vi "WaveSynthV2.vi"(6 "error in":errorcluster) -> (0 "Waves per Pixel":u32, 1 "Delay bw Waves [cycles]":u16, 2 "Sampling Frequency (Hz)":u64, 3 "Waveform":cluster{"tv":dbl[], "DAC Codes":u16[]}, 4 "error out":errorcluster)   [LabVIEW 2018]
uses:
  Controls/WaveFormsAvailable.ctl
  <vilib>/Utility/file.llb/Read Delimited Spreadsheet (DBL).vi
  <vilib>/Utility/file.llb/Write Delimited Spreadsheet (DBL).vi
panel:
  in  "Waveform":T1(tab)
  out "Single Wave":cluster{"all rows":dbl[], "Array":u16[]}(graph)
  out "Wave per Pixel":cluster{dbl[], dbl[]}(graph)
  out "DC Offset":dbl
  out "Frequency Response":cluster{dbl[], dbl[]}(graph)
  in  "Tab Control":enum32{"Temp (Future Controls Idea)", "Page 2"}(tab)
  in  "Scale Precision _Scale":i16(slide)=-3 caption="Scale Precision" scale=-3.0..3.0
  in  "Scale JogWheel":i16(knob) scale=0.0..50.0
  in  "Scale Precision _offset":i16(slide) caption="Scale Precision"
  in  "Offset JogWheel":i16(knob) scale=0.0..50.0
  in  "Scale Precision_Phase":i16(slide) caption="Scale Precision" scale=0.0..3.0
  in  "Phase  JogWheel":i16(knob) scale=0.0..50.0
  out "Time Series":dbl[](array[numeric])
  out "Amplitudes":u16[](array[numeric])
  in  "Save Button":bool
  in  "Start Time (us)":dbl format="%#_6p"
  in  "Number of Samples":u32=2048
  in  "Sampling Frequency (Hz)":u64=1250000000 format="%.2p"
  in  "Waves per Pixel":u32=1
  in  "Delay between waves (us)":dbl
  in  "Frequency (Hz)":u64=40000000 format="%.0p"
  in  "Wave":T2=enum."Ricker"
  in  "Reset Button":bool
  in  "Scale Factor":dbl=1.0
  in  "Offset Factor":dbl
  in  "Phase Delay (Samples)":i32
  in  "Done":bool
  # "Waveform Synthesizer"
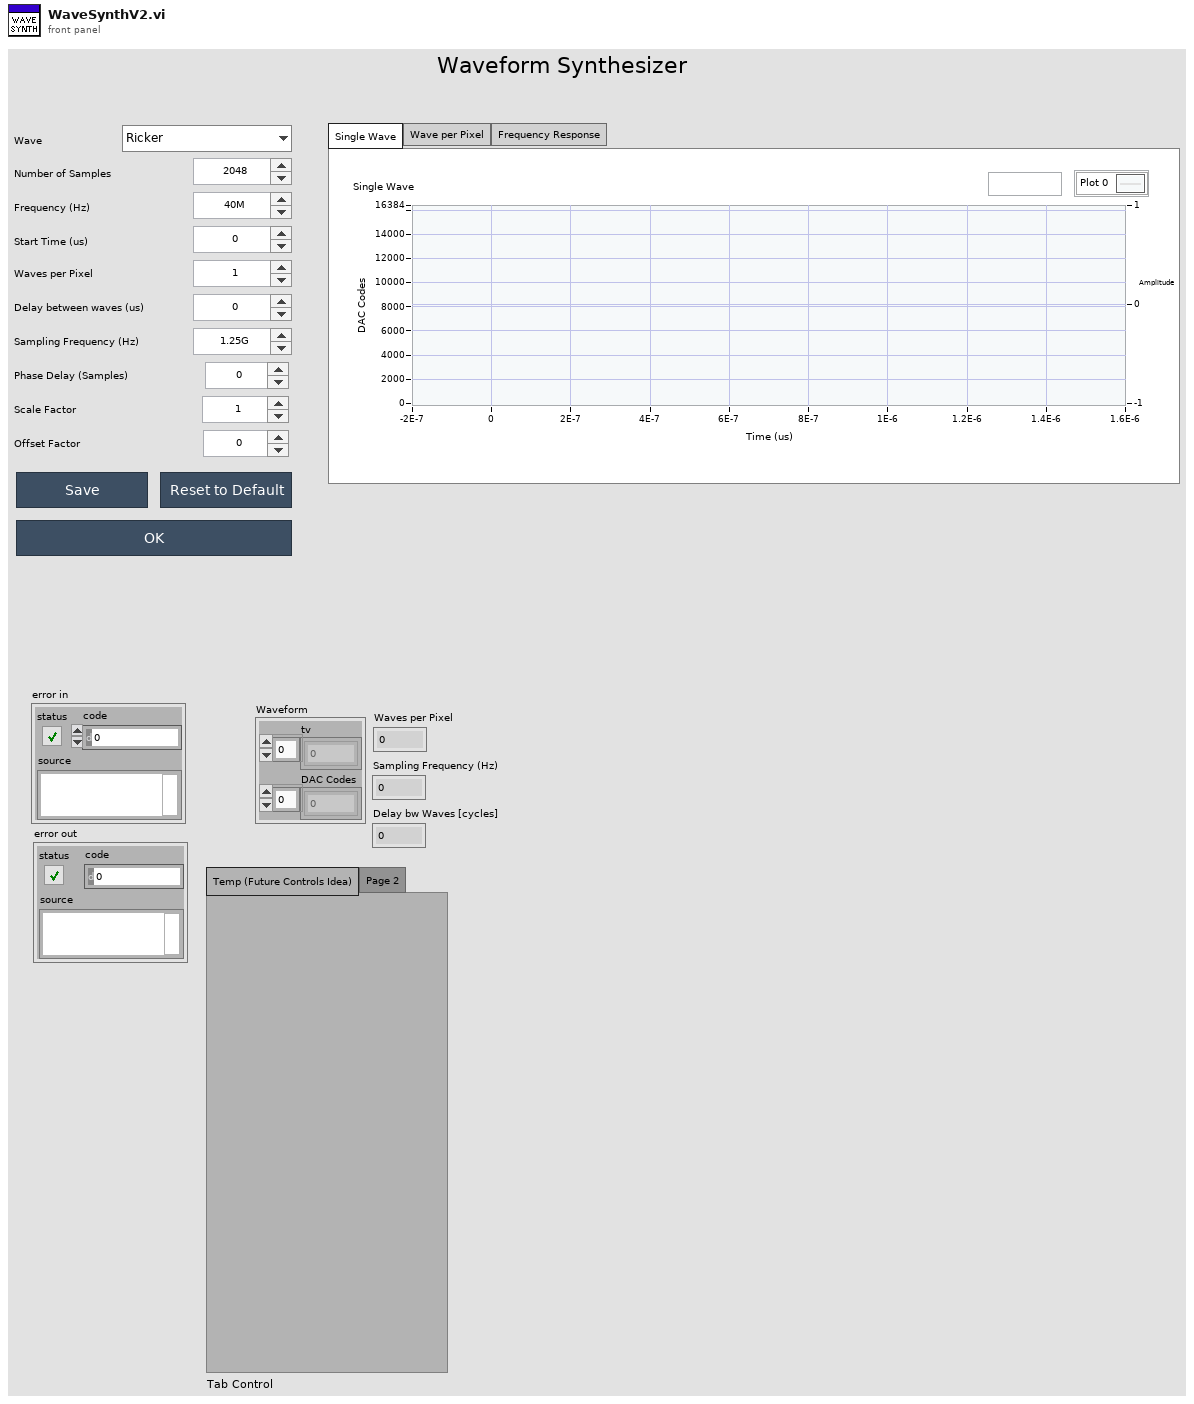
[diagram p1: front panel]
types:
  T1 = enum32{"Single Wave", "Wave per Pixel", "Frequency Response"}
  T2 = typedef "WaveFormsAvailable.ctl" = enum16{"Chirp", "Ricker", "Other..."}
  T3 = enum8{"Enabled", "Disabled", "Disabled and Grayed Out"}
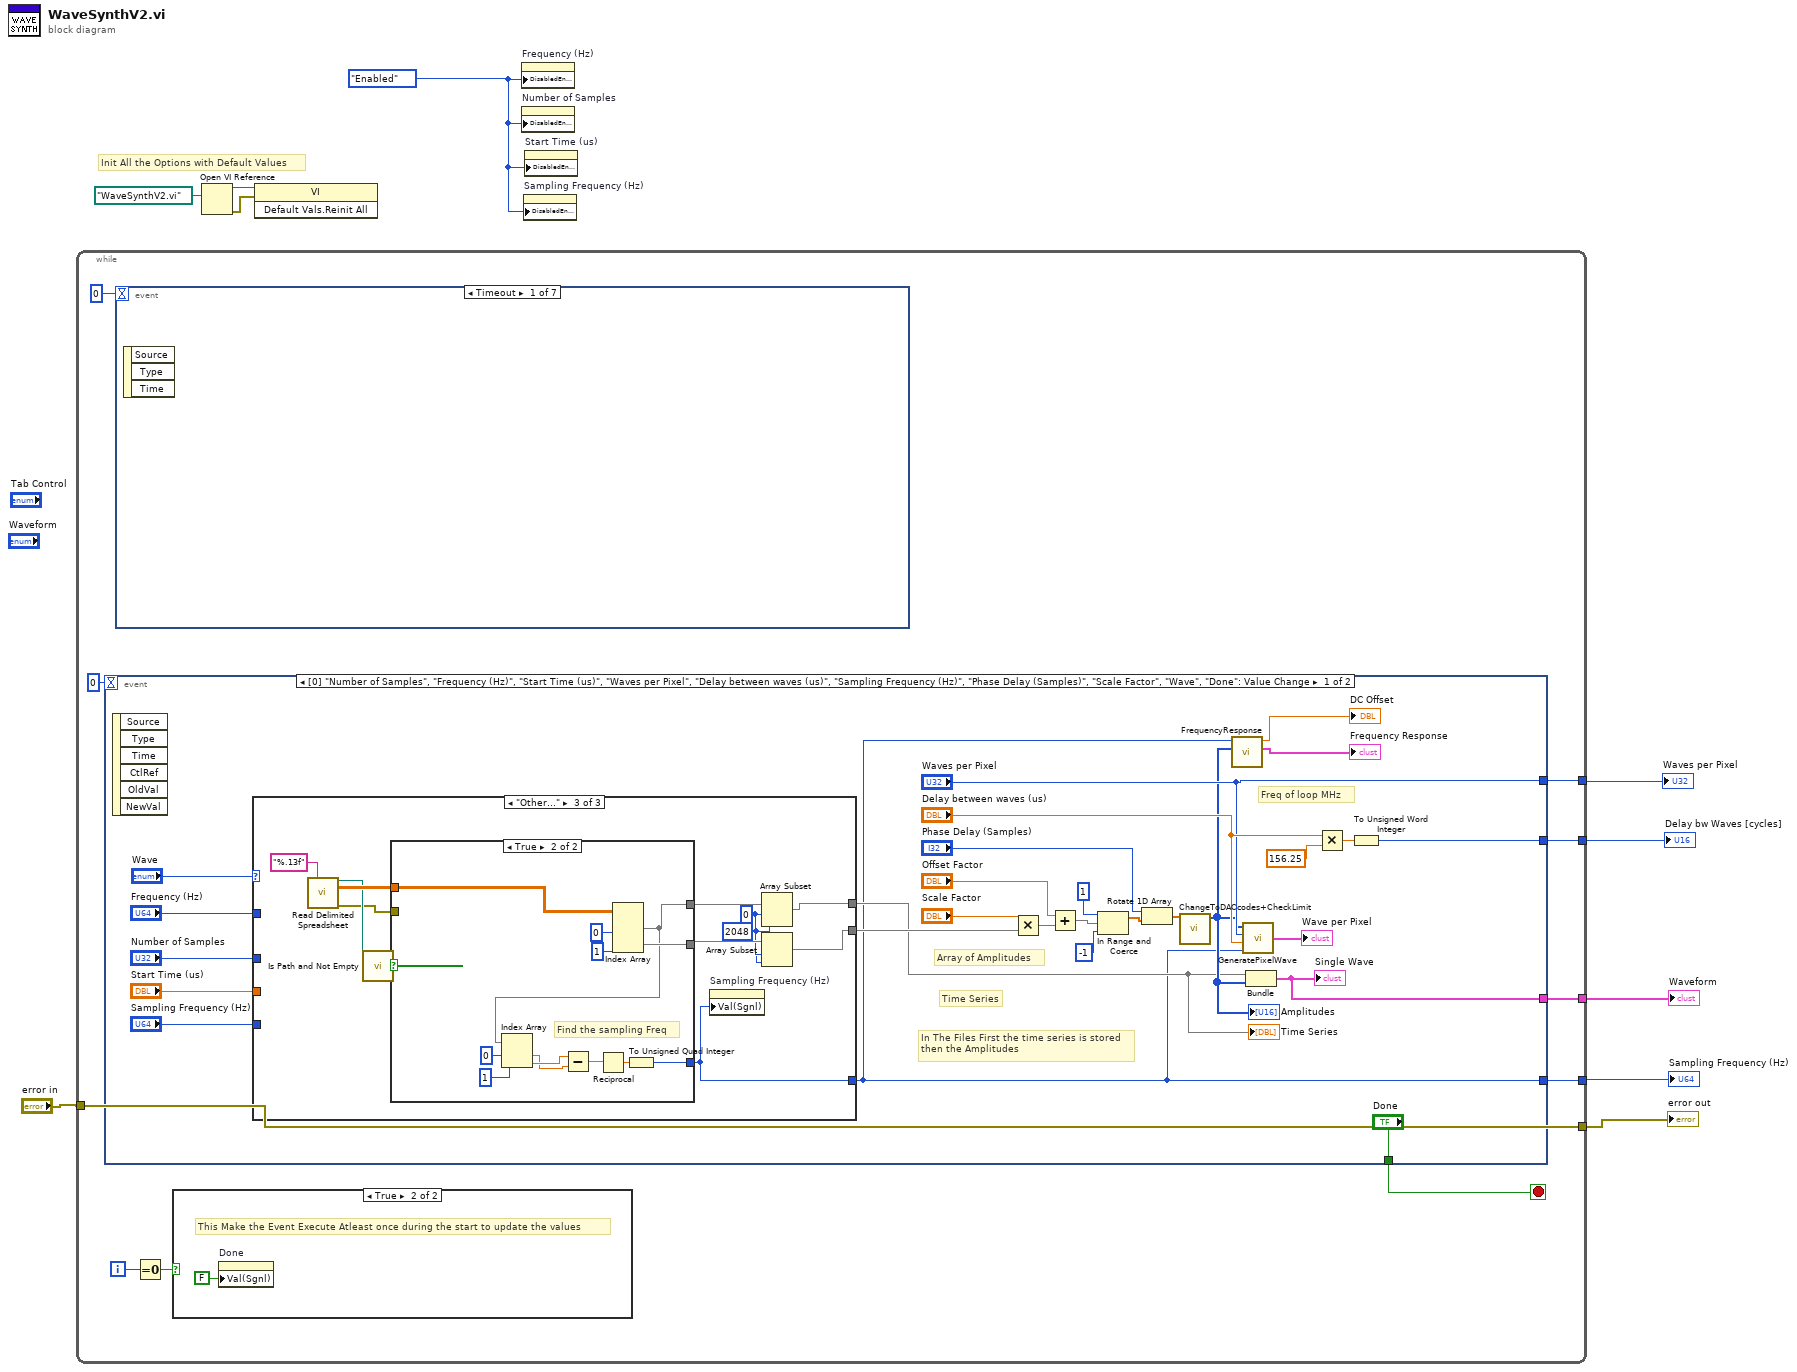
[diagram p0: block diagram]
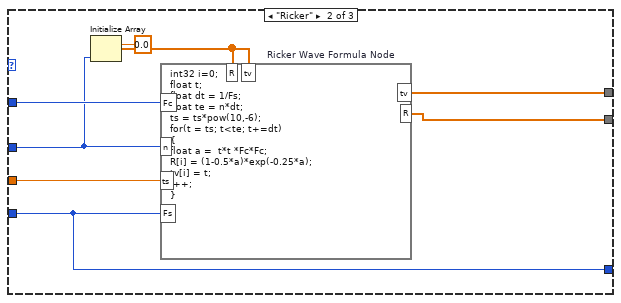
[diagram p4: hidden frame]
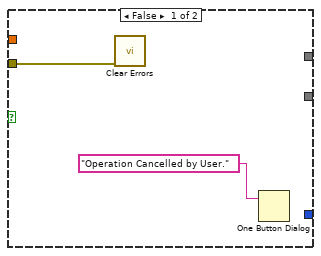
[diagram p5: hidden frame]
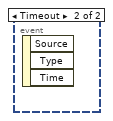
[diagram p6: hidden frame]
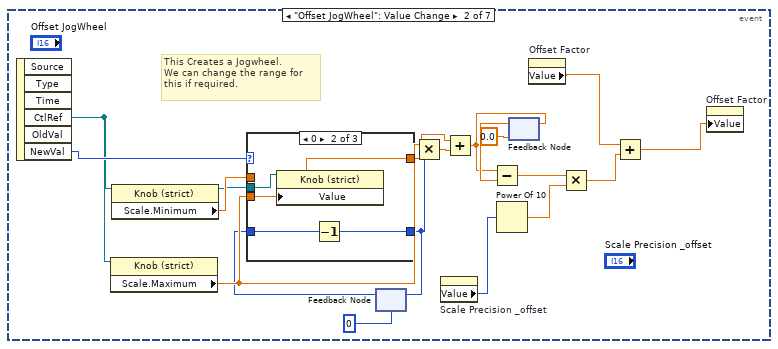
[diagram p7: hidden frame]
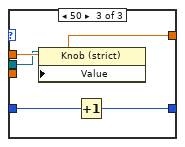
[diagram p9: hidden frame]
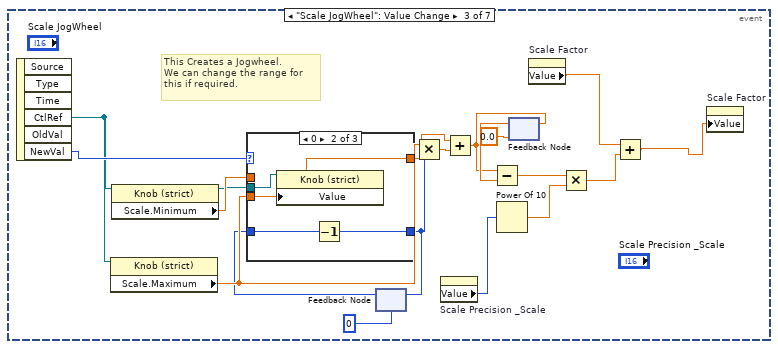
[diagram p10: hidden frame]
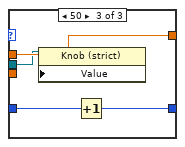
[diagram p12: hidden frame]
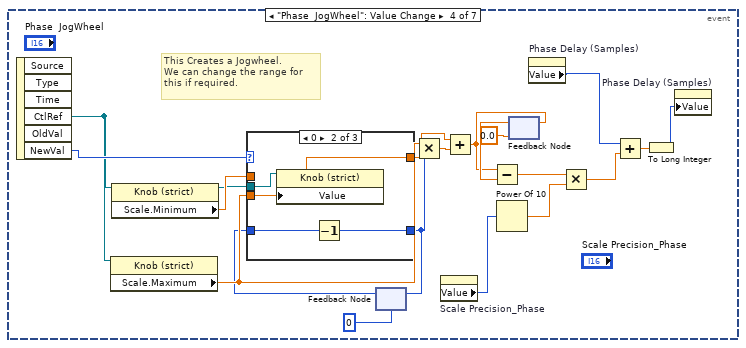
[diagram p13: hidden frame]
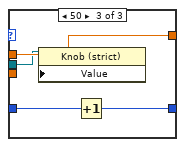
[diagram p15: hidden frame]
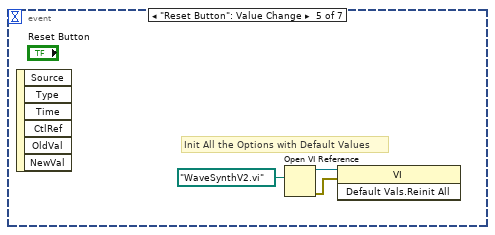
[diagram p16: hidden frame]
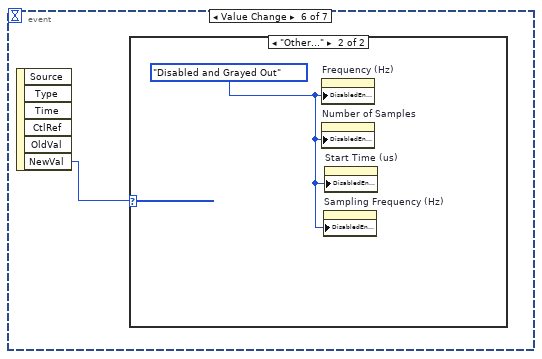
[diagram p17: hidden frame]
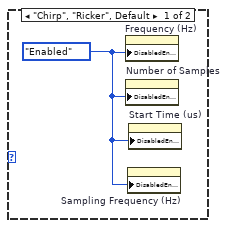
[diagram p18: hidden frame]
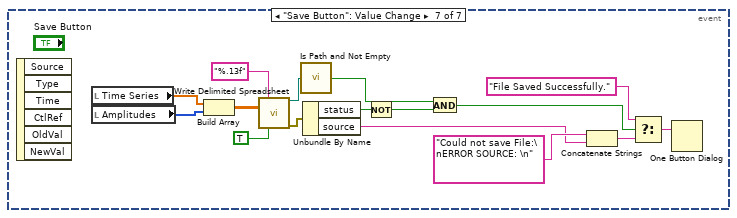
[diagram p19: hidden frame]
diagram:
  w7 = T3."Enabled" ("Disabled")
  # "Init All the Options with Default Values"
  n1 = while {
    tunnel: [w20] -> w6
    tunnel: [w18] -> w5
    tunnel: [w16] -> w4
    tunnel: [w19] -> w3
    tunnel: "error in" -> [w17]
    tunnel: [w17] -> w1
    i -> [w12]
    stop <- w13 stop-if-true
    n2 = event shown="[0] \"Number of Samples\", \"Frequency (Hz)\", \"Start Time (us)\", \"Waves per Pixel\", \"Delay between waves (us)\", \"Sampling Frequency (Hz)\", \"Phase Delay (Samples)\", \"Scale Factor\", \"Wave\", \"Done\": Value Change" {
      selector: _ -> [_ _]
      dyn-events: _ -> [_ _]
      timeout: 0 -> [_ _]
      tunnel: [w36 _] -> w20
      tunnel: ["Waves per Pixel" _] -> w19
      tunnel: [w30 _] -> w18
      tunnel: [w25 _] -> w16
      tunnel: ["Done" _] -> w13
      event "Number of Samples", "Frequency (Hz)", "Start Time (us)", "Waves per Pixel", "Delay between waves (us)", "Sampling Frequency (Hz)", "Phase Delay (Samples)", "Scale Factor", "Done": Value Change {
        # "Freq of loop MHz"
        # "In The Files First the time series is stored \nthen the Amplitudes"
        # "Array of Amplitudes"
        # "Time Series"
        n3 = event-data() -> ()  [unwired: 1 in, 6 out]
        n4 = case shown="\"Other...\"" "Wave" {
          tunnel: [_ w56 w66] -> w26
          tunnel: "Frequency (Hz)" -> [_ w55 _]
          tunnel: "Start Time (us)" -> [_ w54 _]
          tunnel: "Number of Samples" -> [_ w52 _]
          tunnel: [_ w51 w65] -> w28
          tunnel: "Sampling Frequency (Hz)" -> [_ w50 _]
          tunnel: [_ w50 w68] -> w25
          frame "Chirp", Default {
          }
          frame "Ricker" {
            n5 = Initialize Array(0.0 ("element"), w52) -> (w53:dbl[])
            n6 = formula code="int32 i=0;\nfloat t;\nfloat dt = 1/Fs;\nfloat te = n*dt;\nts = ts*pow(10,-6);\nfor(t = ts; t<te; t+=dt)\n{ \nfloat a =  t*t *Fc*Fc;\nR[i] = (1-0.5*a)*exp(-0.25*a);\ntv[i] = t;\ni++;\n}" "Ricker Wave Formula Node"("Fc"=w55, "R"=w53, "ts"=w54, "n"=w52, "Fs"=w50, "tv"=w53) -> ("R"=w51:dbl[], "tv"=w56:dbl[])
          }
          frame "Other..." {
            w62 = 2048 ("length")
            w63 = 0 ("index")
            n7 = call-poly <vilib>:"Read Delimited Spreadsheet.vi"("format (%.3f)"="%.13f" ("format (%d)")) -> ("new file path (Not A Path if cancelled)"=w59:path, "all rows"=w60:dbl[][], "error out"=w58:errorcluster)  [unwired: 9 in, 3 out]
            n8 = call <vilib>:"Is Path and Not Empty.vi"("path"=w59) -> ("Is Path and Not Empty?"=w69:bool)  [unwired: 4 in]
            n9 = case shown="True" w69 {
              tunnel: [_ w80] -> w67
              tunnel: [_ w81] -> w64
              tunnel: [_ w73] -> w68
              tunnel: w60 -> [_ w72]
              tunnel: w58 -> [w71 _]
              frame False {
                n10 = call <vilib>:"Clear Errors.vi"("error in (no error)"=w71) -> ()  [unwired: 5 in, 2 out]
                n11 = One Button Dialog(message="Operation Cancelled by User.") -> ()  [unwired: 1 in, 1 out]
              }
              frame True {
                # "Find the sampling Freq"
                n12 = Index Array(array=w72, index (col) #1=0 ("index (row)"), index (col) #2=1 ("index (col)")) -> (element #1=w80:dbl[], element #2=w81:dbl[])  [unwired: 2 in]
                n13 = Index Array(array=w80, index #1=0 ("index"), index #2=1 ("index")) -> (element #1=w76:dbl, element #2=w77:dbl)
                n14 = Subtract(x=w77, y=w76) -> (x-y=w75:dbl)
                n15 = Reciprocal(x=w75) -> (1/x=w74:dbl)
                n16 = To Unsigned Quad Integer(1:w74) -> (0:w73:u64)
              }
            }
            n17 = property on="Sampling Frequency (Hz)" class="DigNum (strict)"("Val(Sgnl)"=w68) -> ()  [unwired: 2 in, 2 out]
            n18 = Array Subset(array=w67, index=w63, length=w62) -> (w66:dbl[])
            n19 = Array Subset(array=w64, index=w63, length=w62) -> (w65:dbl[])
          }
        }
        "Time Series" <- w26
        n20 = Multiply(x="Scale Factor", y=w28) -> (x*y=w43:dbl[])
        n21 = Add(x="Offset Factor", y=w43) -> (x+y=w39:dbl[])
        n22 = In Range and Coerce(upper limit=1, x=w39, lower limit=-1) -> (coerced(x)=w40:dbl[])  [unwired: 1 out]
        n23 = Rotate 1D Array(1:w40, 2:"Phase Delay (Samples)") -> (0:w27:dbl[])
        n24 = call "ChangeToDACcodes+CheckLimit.vi"("Input Waveform"=w27) -> ("DAC Codes"=w29:u16[])  [unwired: 10 in]
        "Amplitudes" <- w29
        n25 = call "FrequencyResponse.vi"("DAC Codes"=w29, "Sampling Frequency (Hz)"=w25) -> ("Frequency Response"=→"Frequency Response":cluster{dbl[], dbl[]}, "DC Offset"=→"DC Offset":dbl)  [unwired: 8 in]
        n26 = call "GeneratePixelWave.vi"("Fs"=w25, "Delay between waves (us)"="Delay between waves (us)", "Waves per Pixel"="Waves per Pixel", "Single Wave"=w29) -> ("Pixel Wave"=→"Wave per Pixel":cluster{dbl[], "R":dbl[]})
        n27 = Bundle("tv"=w26, "DAC Codes"=w29) -> (w36:cluster{"tv":dbl[], "DAC Codes":u16[]})  [unwired: 1 in]
        "Single Wave" <- w36
        n28 = Multiply(x="Delay between waves (us)", y=156.25) -> (x*y=w31:dbl)
        n29 = To Unsigned Word Integer(number=w31) -> (unsigned 16bit integer=w30:u16)
      }
      event Timeout {
        n30 = event-data() -> ()  [unwired: 1 in, 3 out]
      }
    }
    n31 = event shown="[0] Timeout" {
      selector: _ -> [_ _ _ _ _ _ _]
      dyn-events: _ -> [_ _ _ _ _ _ _]
      timeout: 0 -> [_ _ _ _ _ _ _]
      event Timeout {
        n32 = event-data() -> ()  [unwired: 1 in, 3 out]
      }
      event "Offset JogWheel": Value Change {
        # "This Creates a Jogwheel.\nWe can change the range for \nthis if required."
        n33 = event-data() -> ("CtlRef"=w86:refnum<vi>, "NewVal"=w87:i16)  [unwired: 1 in, 4 out]
        n34 = property on="Property Node" class="Knob (strict)"(reference=w86) -> ("Scale.Maximum"=w100:dbl)  [unwired: 1 in, 2 out]
        n35 = property on="Property Node" class="Knob (strict)"(reference=w86) -> (reference out=w85:refnum<vi>, "Scale.Minimum"=w99:dbl)  [unwired: 1 in, 1 out]
        n36 = feedback #1(0) -> (w88:i32)
        n37 = case shown="0" w87 {
          selector: w87 -> [w104 _ _]
          tunnel: w100 -> [_ w108 _]
          tunnel: w99 -> [_ _ w112]
          tunnel: [w104 w108 w112] -> w102
          tunnel: [w103 w107 w110] -> w89
          tunnel: w88 -> [w103 w106 w111]
          tunnel: w85 -> [_ w105 w109]
          frame Default {
          }
          frame 0 {
            n38 = property on="Property Node" class="Knob (strict)"(reference=w105, "Value"=w108) -> ()  [unwired: 1 in, 2 out]
            n39 = Decrement(x=w106) -> (x-1=w107:i32)
          }
          frame 50 {
            n40 = property on="Property Node" class="Knob (strict)"(reference=w109, "Value"=w112) -> ()  [unwired: 1 in, 2 out]
            n41 = Increment(x=w111) -> (x+1=w110:i32)
          }
        }
        n42 = feedback-in #1(w89) -> ()
        n43 = Multiply(x=w100, y=w89) -> (x*y=w101:dbl)
        n44 = property on="Scale Precision _offset" class="Slide (strict)"() -> ("Value"=w98:i16)  [unwired: 2 in, 2 out]
        n45 = Add(x=w102, y=w101) -> (x+y=w92:dbl)
        n46 = Power Of 10(x=w98) -> (10^x=w94:dbl)
        n47 = feedback #2(0.0) -> (w96:dbl)
        n48 = Subtract(x=w92, y=w96) -> (x-y=w97:dbl)
        n49 = feedback-in #2(w92) -> ()
        n50 = property on="Offset Factor" class="DigNum (strict)"() -> ("Value"=w91:dbl)  [unwired: 2 in, 2 out]
        n51 = Multiply(x=w97, y=w94) -> (x*y=w95:dbl)
        n52 = Add(x=w91, y=w95) -> (x+y=w84:dbl)
        n53 = property on="Offset Factor" class="DigNum (strict)"("Value"=w84) -> ()  [unwired: 2 in, 2 out]
      }
      event "Scale JogWheel": Value Change {
        # "This Creates a Jogwheel.\nWe can change the range for \nthis if required."
        n54 = event-data() -> ("CtlRef"=w115:refnum<vi>, "NewVal"=w116:i16)  [unwired: 1 in, 4 out]
        n55 = property on="Property Node" class="Knob (strict)"(reference=w115) -> ("Scale.Maximum"=w129:dbl)  [unwired: 1 in, 2 out]
        n56 = property on="Property Node" class="Knob (strict)"(reference=w115) -> (reference out=w114:refnum<vi>, "Scale.Minimum"=w128:dbl)  [unwired: 1 in, 1 out]
        n57 = feedback #3(0) -> (w117:i32)
        n58 = case shown="0" w116 {
          selector: w116 -> [w133 _ _]
          tunnel: w129 -> [_ w137 _]
          tunnel: w128 -> [_ _ w141]
          tunnel: [w133 w137 w141] -> w131
          tunnel: [w132 w136 w139] -> w118
          tunnel: w117 -> [w132 w135 w140]
          tunnel: w114 -> [_ w134 w138]
          frame Default {
          }
          frame 0 {
            n59 = property on="Property Node" class="Knob (strict)"(reference=w134, "Value"=w137) -> ()  [unwired: 1 in, 2 out]
            n60 = Decrement(x=w135) -> (x-1=w136:i32)
          }
          frame 50 {
            n61 = property on="Property Node" class="Knob (strict)"(reference=w138, "Value"=w141) -> ()  [unwired: 1 in, 2 out]
            n62 = Increment(x=w140) -> (x+1=w139:i32)
          }
        }
        n63 = feedback-in #3(w118) -> ()
        n64 = Multiply(x=w129, y=w118) -> (x*y=w130:dbl)
        n65 = property on="Scale Precision _Scale" class="Slide (strict)"() -> ("Value"=w127:i16)  [unwired: 2 in, 2 out]
        n66 = Add(x=w131, y=w130) -> (x+y=w121:dbl)
        n67 = Power Of 10(x=w127) -> (10^x=w123:dbl)
        n68 = feedback #4(0.0) -> (w125:dbl)
        n69 = Subtract(x=w121, y=w125) -> (x-y=w126:dbl)
        n70 = feedback-in #4(w121) -> ()
        n71 = property on="Scale Factor" class="DigNum (strict)"() -> ("Value"=w120:dbl)  [unwired: 2 in, 2 out]
        n72 = Multiply(x=w126, y=w123) -> (x*y=w124:dbl)
        n73 = Add(x=w120, y=w124) -> (x+y=w113:dbl)
        n74 = property on="Scale Factor" class="DigNum (strict)"("Value"=w113) -> ()  [unwired: 2 in, 2 out]
      }
      event "Phase  JogWheel": Value Change {
        # "This Creates a Jogwheel.\nWe can change the range for \nthis if required."
        n75 = event-data() -> ("CtlRef"=w143:refnum<vi>, "NewVal"=w144:i16)  [unwired: 1 in, 4 out]
        n76 = property on="Property Node" class="Knob (strict)"(reference=w143) -> ("Scale.Maximum"=w159:dbl)  [unwired: 1 in, 2 out]
        n77 = property on="Property Node" class="Knob (strict)"(reference=w143) -> (reference out=w142:refnum<vi>, "Scale.Minimum"=w158:dbl)  [unwired: 1 in, 1 out]
        n78 = feedback #5(0) -> (w145:i32)
        n79 = case shown="0" w144 {
          selector: w144 -> [w163 _ _]
          tunnel: w159 -> [_ w167 _]
          tunnel: w158 -> [_ _ w171]
          tunnel: [w163 w167 w171] -> w161
          tunnel: [w162 w166 w169] -> w146
          tunnel: w145 -> [w162 w165 w170]
          tunnel: w142 -> [_ w164 w168]
          frame Default {
          }
          frame 0 {
            n80 = property on="Property Node" class="Knob (strict)"(reference=w164, "Value"=w167) -> ()  [unwired: 1 in, 2 out]
            n81 = Decrement(x=w165) -> (x-1=w166:i32)
          }
          frame 50 {
            n82 = property on="Property Node" class="Knob (strict)"(reference=w168, "Value"=w171) -> ()  [unwired: 1 in, 2 out]
            n83 = Increment(x=w170) -> (x+1=w169:i32)
          }
        }
        n84 = feedback-in #5(w146) -> ()
        n85 = Multiply(x=w159, y=w146) -> (x*y=w160:dbl)
        n86 = property on="Scale Precision_Phase" class="Slide (strict)"() -> ("Value"=w157:i16)  [unwired: 2 in, 2 out]
        n87 = Add(x=w161, y=w160) -> (x+y=w151:dbl)
        n88 = Power Of 10(x=w157) -> (10^x=w153:dbl)
        n89 = feedback #6(0.0) -> (w155:dbl)
        n90 = Subtract(x=w151, y=w155) -> (x-y=w156:dbl)
        n91 = feedback-in #6(w151) -> ()
        n92 = property on="Phase Delay (Samples)" class="DigNum (strict)"() -> ("Value"=w150:i32)  [unwired: 2 in, 2 out]
        n93 = Multiply(x=w156, y=w153) -> (x*y=w154:dbl)
        n94 = Add(x=w150, y=w154) -> (x+y=w149:dbl)
        n95 = To Long Integer(number=w149) -> (32bit integer=w148:i32)
        n96 = property on="Phase Delay (Samples)" class="DigNum (strict)"("Value"=w148) -> ()  [unwired: 2 in, 2 out]
      }
      event "Reset Button": Value Change {
        # "Init All the Options with Default Values"
        n97 = event-data() -> ()  [unwired: 1 in, 6 out]
        n98 = Open VI Reference(vi path=path "WaveSynthV2.vi") -> (vi reference=w173:refnum<vi>, error out=w174:errorcluster)  [unwired: 5 in]
        n99 = invoke class="VI" method="Default Vals.Reinit All"(reference=w173, error in=w174) -> ()  [unwired: 1 in, 3 out]
      }
      event Value Change {
        n100 = event-data() -> ("NewVal"=w175:T2)  [unwired: 1 in, 5 out]
        n101 = case shown="\"Other...\"" w175 {
          frame "Chirp", "Ricker", Default {
            w176 = T3."Enabled" ("Disabled")
            n102 = property on="Frequency (Hz)" class="DigNum (strict)"("DisabledEnum"=w176) -> ()  [unwired: 2 in, 2 out]
            n103 = property on="Number of Samples" class="DigNum (strict)"("DisabledEnum"=w176) -> ()  [unwired: 2 in, 2 out]
            n104 = property on="Sampling Frequency (Hz)" class="DigNum (strict)"("DisabledEnum"=w176) -> ()  [unwired: 2 in, 2 out]
            n105 = property on="Start Time (us)" class="DigNum (strict)"("DisabledEnum"=w176) -> ()  [unwired: 2 in, 2 out]
          }
          frame "Other..." {
            w177 = T3."Disabled and Grayed Out" ("Disabled")
            n106 = property on="Frequency (Hz)" class="DigNum (strict)"("DisabledEnum"=w177) -> ()  [unwired: 2 in, 2 out]
            n107 = property on="Number of Samples" class="DigNum (strict)"("DisabledEnum"=w177) -> ()  [unwired: 2 in, 2 out]
            n108 = property on="Sampling Frequency (Hz)" class="DigNum (strict)"("DisabledEnum"=w177) -> ()  [unwired: 2 in, 2 out]
            n109 = property on="Start Time (us)" class="DigNum (strict)"("DisabledEnum"=w177) -> ()  [unwired: 2 in, 2 out]
          }
        }
      }
      event "Save Button": Value Change {
        n110 = event-data() -> ()  [unwired: 1 in, 6 out]
        n111 = local read "Time Series"() -> (w180:dbl[])
        n112 = local read "Amplitudes"() -> (w179:u16[])
        n113 = Build Array(w180, w179) -> (w193:dbl[][])
        n114 = call-poly <vilib>:"Write Delimited Spreadsheet.vi"("format (%.3f)"="%.13f", "2D data"=w193, "transpose? (no:F)"=TRUE) -> ("new file path (Not A Path if cancelled)"=w185:path, "error out"=w189:errorcluster)  [unwired: 11 in]
        n115 = call <vilib>:"Is Path and Not Empty.vi"("path"=w185) -> ("Is Path and Not Empty?"=w183:bool)  [unwired: 4 in]
        n116 = Unbundle By Name(w189) -> ("status"=w184:bool, "source"=w186:string)
        n117 = Not(x=w184) -> (.not. x?=w181:bool)
        n118 = And(x=w183, y=w181) -> (x .and. y?=w182:bool)
        n119 = Concatenate Strings("Could not save File:\nERROR SOURCE: \n", w186) -> (w187:string)
        n120 = Select(t="File Saved Successfully.", s=w182, f=w187) -> (s? t:f=w191:string)
        n121 = One Button Dialog(message=w191) -> ()  [unwired: 1 in, 1 out]
      }
    }
    n122 = Equal To 0?(x=w12) -> (x = 0?=w11:bool)
    n123 = case shown="True" w11 {
      frame False {
      }
      frame True {
        # "This Make the Event Execute Atleast once during the start to update the values"
        n124 = property on="Done" class="Bool (strict)"("Val(Sgnl)"=FALSE ("Value (Signaling)")) -> ()  [unwired: 2 in, 2 out]
      }
    }
  }
  "Waveform" <- w6
  "Delay bw Waves [cycles]" <- w5
  "Sampling Frequency (Hz)" <- w4
  "Waves per Pixel" <- w3
  "error out" <- w1
  n125 = Open VI Reference(vi path=path "WaveSynthV2.vi") -> (vi reference=w9:refnum<vi>, error out=w8:errorcluster)  [unwired: 5 in]
  n126 = invoke class="VI" method="Default Vals.Reinit All"(reference=w9, error in=w8) -> ()  [unwired: 1 in, 3 out]
  n127 = property on="Frequency (Hz)" class="DigNum (strict)"("DisabledEnum"=w7) -> ()  [unwired: 2 in, 2 out]
  n128 = property on="Number of Samples" class="DigNum (strict)"("DisabledEnum"=w7) -> ()  [unwired: 2 in, 2 out]
  n129 = property on="Sampling Frequency (Hz)" class="DigNum (strict)"("DisabledEnum"=w7) -> ()  [unwired: 2 in, 2 out]
  n130 = property on="Start Time (us)" class="DigNum (strict)"("DisabledEnum"=w7) -> ()  [unwired: 2 in, 2 out]
